vi "Get Key For Phrase.vi"(8 "error in":errorcluster, 9 "Target Language (current lang)":string, 10 "Phrase":string) -> (0 "error out":errorcluster, 2 "Key":string)   [LabVIEW 2020]
doc: "Gets the localized phrase by key from the current dictionary.\n\nKey: Unique identifier defined in the dictionary\nTarget Language (current lang): Optional input. Set this to translate a phase to a language other than the current language."
uses:
  SubVIs/Localization FGV Action -- Enum.ctl
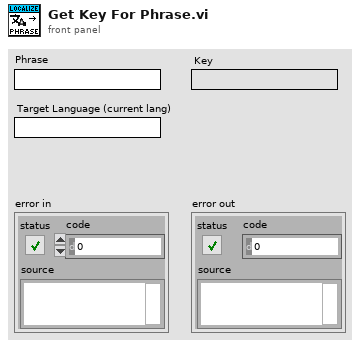
[diagram p1: front panel]
types:
  T1 = typedef "Localization FGV Action -- Enum.ctl" = enum16{"Read Dictionary", "Translate VIs", "Register VI", "Get Languages", "Translate Phrase", "Get Key For Phrase", "Get Phrase For Phrase", "Translate VI", "Unregister"}
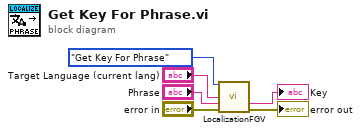
[diagram p0: block diagram]
diagram:
  n1 = call "LocalizationFGV.vi"("Action"=Localization_FGV_Action_--_Enum."Get Key For Phrase", "Target Language"="Target Language (current lang)", "Input"="Phrase", "error in"="error in") -> ("Result"=→"Key":string, "error out"=→"error out":errorcluster)  [unwired: 6 in, 4 out]
